vi "Function Gen Scan.vi"(8 "error in (no error)":errorcluster, 10 "Function Generator.lvclass":refnum<class "Function Generator.lvclass">, 11 "Function Gen Scan in":refnum<class "Function Gen Scan.lvclass">) -> (0 "error out":errorcluster, 3 "Function Gen Scan out":refnum<class "Function Gen Scan.lvclass">)   [LabVIEW 2009, in "Function Gen Scan.lvclass"]
uses:
  Function Gen Scan.lvclass
  Instruments/Function Generator/Function Generator.lvclass
  Scanner/Scanner.lvclass
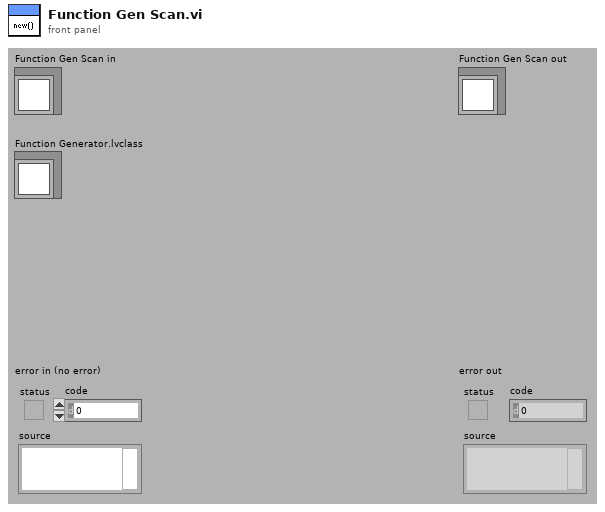
[diagram p1: front panel]
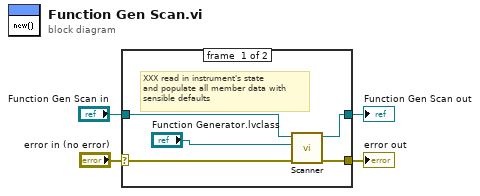
[diagram p0: block diagram]
diagram:
  n1 = case shown="No Error" "error in (no error)" {
    selector: "error in (no error)" -> [w7 w11]
    tunnel: [w6 w11] -> w3
    tunnel: [w8 w10] -> w1
    tunnel: "Function Gen Scan in" -> [w9 w10]
    frame #0 {
      # "XXX read in instrument's state\nand populate all member data with\nsensible defaults"
      n2 = call "Scanner.vi"("error in (no error)"=w7, "Scannable"="Function Generator.lvclass", "Scanner.lvclass in"=w9) -> ("error out"=w6:errorcluster, "Scanner.lvclass out"=w8:refnum<class "Function Gen Scan.lvclass">)  [unwired: 1 in, 6 out]
    }
    frame #1 {
    }
  }
  "error out" <- w3
  "Function Gen Scan out" <- w1
